vi "calc_DOM_min.vi"(11 "Input RowData":T1) -> (3 "DOM":dbl)   [LabVIEW 2019]
uses:
  RowData_Type.ctl
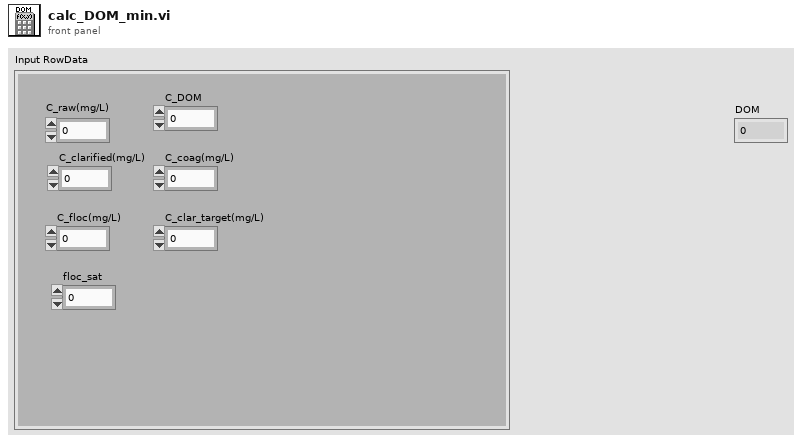
[diagram p1: front panel]
types:
  T1 = typedef "RowData_Type.ctl" = cluster{"C_raw(mg/L)":dbl, "C_clarified(mg/L)":dbl, "C_floc(mg/L)":dbl, "floc_sat":dbl, "C_DOM":dbl, "C_coag(mg/L)":dbl, "C_clar_target(mg/L)":dbl}
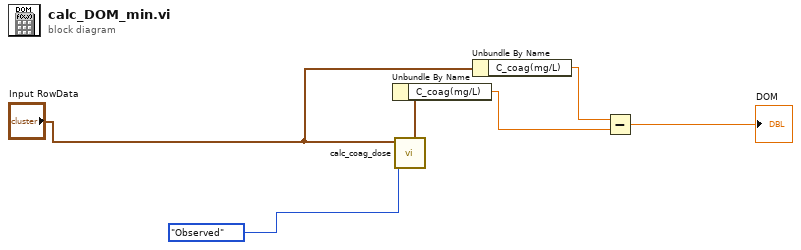
[diagram p0: block diagram]
diagram:
  n1 = call "calc_coag_dose.vi"("Enum"=enum16{"Observed", "Target"}."Observed", "RowData input"="Input RowData") -> ("RowData output"=w4:T1)  [unwired: 9 in]
  n2 = Unbundle By Name(w4) -> ("C_coag(mg/L)"=w1:dbl)
  n3 = Unbundle By Name("Input RowData") -> ("C_coag(mg/L)"=w2:dbl)
  n4 = Subtract(x=w2, y=w1) -> (x-y=→"DOM":dbl)
